vi "Write Signals to Monitor.vi"(8 "error in (no error)":errorcluster, 10 "data value":string[][](array[string]), 11 "Performanced XNET CAN Signal Logger in":refnum<class "Performanced XNET CAN Signal Logger.lvclass">) -> (0 "error out":errorcluster, 3 "Performanced XNET CAN Signal Logger out":refnum<class "Performanced XNET CAN Signal Logger.lvclass">)   [LabVIEW 2021, in "Performanced XNET CAN Signal Logger.lvlib" / "Performanced XNET CAN Signal Logger.lvclass"]
uses:
  Performanced XNET CAN Signal Logger.lvclass
  Performanced XNET CAN Signal Logger.lvclass/Performanced XNET CAN Signal Logger.ctl
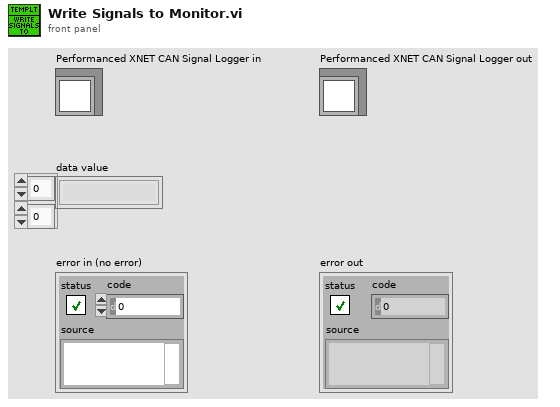
[diagram p1: front panel]
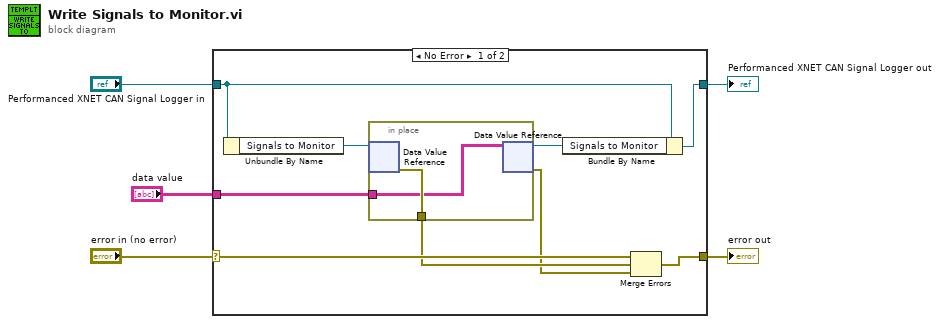
[diagram p0: block diagram]
diagram:
  n1 = case shown="No Error" "error in (no error)" {
    selector: "error in (no error)" -> [w14 w17]
    tunnel: [w8 w17] -> w4
    tunnel: [w13 w18] -> w2
    tunnel: "Performanced XNET CAN Signal Logger in" -> [w12 w18]
    tunnel: "data value" -> [w9 _]
    frame No Error {
      n2 = Unbundle By Name(w12) -> ("Signals to Monitor"=w11:refnum<data-value>)
      n3 = in-place {
        in-place-border: [w16] -> w7
        in-place-border: w9 -> [w15]
        n4 = in-place-dvr #1(w11) -> (w16:errorcluster)  [unwired: 1 out]
        n5 = in-place-dvr #1(w15) -> (w10:refnum<data-value>, w6:errorcluster)
      }
      n6 = Bundle By Name(cluster=w12, "Signals to Monitor"=w10) -> (w13:refnum<class "Performanced XNET CAN Signal Logger.lvclass">)
      n7 = Merge Errors(w14, w7, w6) -> (w8:errorcluster)
    }
    frame Error {
    }
  }
  "error out" <- w4
  "Performanced XNET CAN Signal Logger out" <- w2
